vi "ApplyDeadband.vi"(10 "Deadband":dbl, 11 "Value":dbl) -> (3 "Value`":dbl)   [LabVIEW 2012]
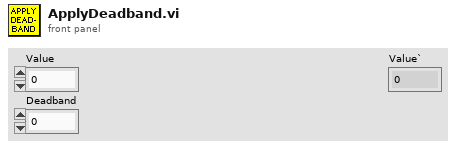
[diagram p1: front panel]
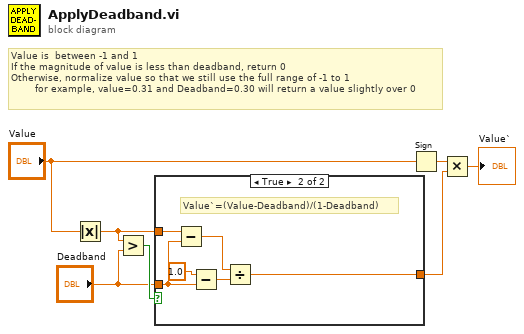
[diagram p0: block diagram]
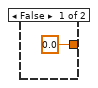
[diagram p2: hidden frame]
diagram:
  # "Value is  between -1 and 1\nIf the magnitude of value is less than deadband, return 0\nOtherwise, normalize value so that we still use the full range of -1 to 1\n        for example, value=0.31 and Deadband=0.30 will return a value slightly over 0"
  n1 = Absolute Value(x="Value") -> (abs(x)=w5:dbl)
  n2 = Greater?(x=w5, y="Deadband") -> (0:w7:bool)
  n3 = case shown="True" w7 {
    tunnel: "Deadband" -> [_ w10]
    tunnel: w5 -> [_ w14]
    tunnel: [0.0 w9] -> w4
    frame False {
    }
    frame True {
      # "Value`=(Value-Deadband)/(1-Deadband)"
      n4 = Subtract(x=w14, y=w10) -> (x-y=w13:dbl)
      n5 = Subtract(x=1.0, y=w10) -> (x-y=w12:dbl)
      n6 = Divide(x=w13, y=w12) -> (x/y=w9:dbl)
    }
  }
  n7 = Sign(1:"Value") -> (0:w3:dbl)
  n8 = Multiply(x=w3, y=w4) -> (x*y=→"Value`":dbl)
